vi "Wait for Device Ready.vi"(4 "stop notifier ref (none)":refnum<notifier>, 6 "stop ref (none)":refnum<vi>, 8 "error in":errorcluster, 10 "timeout [s] (5s)":dbl=5.0, 11 "VISA resource in":refnum<visa-resource-name>) -> (0 "error out":errorcluster, 2 "was aborted?":bool, 3 "VISA resource out":refnum<visa-resource-name>)   [LabVIEW 2013, in "3458A Virtual Digitizer.lvlib" / "3458A Digitizing Low Levels.lvlib"]
doc: "This VI checks device ready flag in the STB. The waiting has timeout option. When timeout is reached it will generate error. It can be also terminated by reference to boolean variable, i.e. if the variable is True. Another way to terminate it is boolean notifier. If the notification is detected and the message content is True it terminates the wait loop.\nIf the waiting was aborted by timeout or stop or error it will return True at 'was aborted?' output.\n\nNote: Reentrant VI so it can be executed in parallel for multiple 3458A sessions."
uses:
  3458A Digitizing Low Levels.lvlib
  <vilib>/Utility/error.llb/Error Cluster From Error Code.vi
  <vilib>/ErrorRing/Error Ring.xnode
  3458A Basic Driver/3458A Basic Driver.lvlib
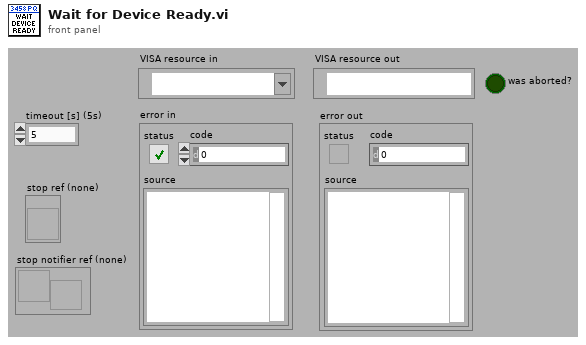
[diagram p1: front panel]
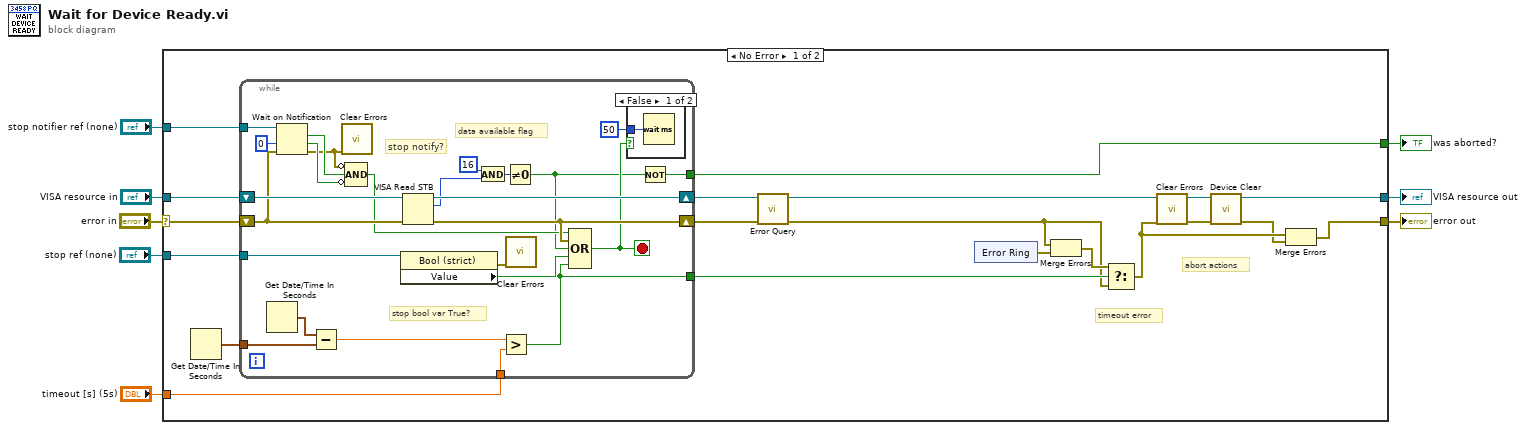
[diagram p0: block diagram]
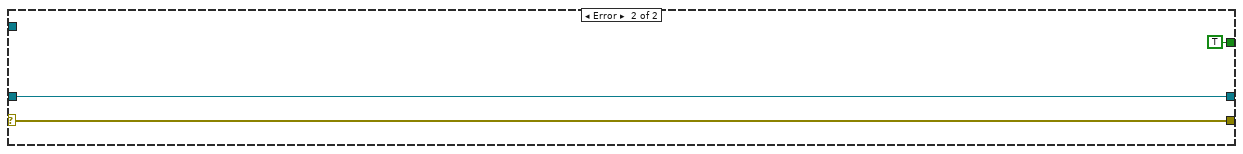
[diagram p3: hidden frame]
diagram:
  n1 = case shown="No Error" "error in" {
    selector: "error in" -> [w25 w61]
    tunnel: [w16 w61] -> w6
    tunnel: "VISA resource in" -> [w27 w60]
    tunnel: [w13 w60] -> w5
    tunnel: "stop ref (none)" -> [w26 _]
    tunnel: "timeout [s] (5s)" -> [w23 _]
    tunnel: "stop notifier ref (none)" -> [w19 _]
    tunnel: [w15 TRUE] -> w1
    frame No Error {
      # "abort actions"
      # "timeout error"
      n2 = Get Date/Time In Seconds() -> (seconds since 1Jan1904=w24:timestamp)
      n3 = while {
        shift-right: [w53] -> w12
        shift-left: w25 -> [w41]
        shift-right: [w56] -> w11
        shift-left: w27 -> [w57]
        tunnel: w26 -> [w51]
        tunnel: w24 -> [w44]
        tunnel: w23 -> [w45]
        tunnel: [w42] -> w22
        tunnel: w19 -> [w40]
        tunnel: [w34] -> w15
        stop <- w47 stop-if-true
        # "stop bool var True?"
        # "stop notify?"
        # "data available flag"
        n4 = Get Date/Time In Seconds() -> (seconds since 1Jan1904=w43:timestamp)
        n5 = Wait on Notification(notifier=w40, timeout in ms (-1)=0, error in (no error)=w41) -> (notification=w38:bool, timed out?=w39:bool, error out=w37:errorcluster)  [unwired: 1 in, 1 out]
        n6 = Subtract(x=w43, y=w44) -> (x-y=w46:dbl)
        n7 = call <vilib>:"Clear Errors.vi"("error in (no error)"=w37) -> ()  [unwired: 6 in, 1 out]
        n8 = Compound Arithmetic op=AND(invert w37, w38, invert w39) -> (w36:bool)
        n9 = property class="Bool (strict)"(reference=w51) -> (error out=w49:errorcluster, "Value"=w50:bool)  [unwired: 1 in, 1 out]
        n10 = VISA Read STB(8:w41, 11:w57) -> (0:w53:errorcluster, 2:w55:u16, 3:w56:refnum<visa-resource-name>)
        n11 = And(x=u16 16, y=w55) -> (x .and. y?=w52:u16)
        n12 = Greater?(x=w46, y=w45) -> (0:w42:bool)
        n13 = Not Equal To 0?(x=w52) -> (x != 0?=w35:bool)
        n14 = call <vilib>:"Clear Errors.vi"("error in (no error)"=w49) -> ()  [unwired: 6 in, 1 out]
        n15 = Compound Arithmetic op=OR(w36, w53, w35, w50, w42) -> (w47:bool)
        n16 = case shown="False" w47 {
          tunnel: u32 50 ("milliseconds to wait") -> [w58 _]
          frame False {
            n17 = Wait (ms)(milliseconds to wait=w58) -> ()  [unwired: 1 out]
          }
          frame True {
          }
        }
        n18 = Not(x=w35) -> (.not. x?=w34:bool)
      }
      n19 = call "Error Query.vi"("error in (no error)"=w12, "VISA resource name"=w11) -> ("error out"=w9:errorcluster, "VISA resource name out"=w10:refnum<visa-resource-name>)  [unwired: 6 in, 2 out]
      n20 = xnode "Error Ring"() -> ("error out"=w21:errorcluster)
      n21 = Merge Errors(w9, w21) -> (w20:errorcluster)
      n22 = Select(t=w20, s=w22, f=w9) -> (s? t:f=w17:errorcluster)
      n23 = call <vilib>:"Clear Errors.vi"("error in (no error)"=w17) -> ("error out"=w18:errorcluster)  [unwired: 6 in]
      n24 = call "Device Clear.vi"("error in(no error)"=w18, "VISA Resource Name"=w10) -> ("error out"=w14:errorcluster, "VISA resource name out"=w13:refnum<visa-resource-name>)  [unwired: 8 in]
      n25 = Merge Errors(w17, w14) -> (w16:errorcluster)
    }
    frame Error {
    }
  }
  "VISA resource out" <- w5
  "error out" <- w6
  "was aborted?" <- w1
